vi "MonoSpec50 Goto.vi"(4 "PosDem":dbl caption="Position\nDemandée (nm)", 5 "Abort Ref":refnum<vi>, 6 "error in (no error)":errorcluster, 7 "PosAct":dbl caption="Position\nActuelle (nm)", 8 "Moving Ref":refnum<vi>, 9 "Ask Act Pos":bool=TRUE caption="Demander la \nposition actuelle (nm)") -> (0 "error out":errorcluster, 1 "PosAct Out":dbl caption="Position\nActuelle (nm)")   [LabVIEW 2012]
doc: "Ce Vi permet l'envoie de commande de déplacement au contrôlleur de moteur du monochromateur MonoSpec50."
uses:
  <userlib>/Monospec 50/MonoSpec50 Goto States.ctl
panel:
  out "large":bool
  out "NegPulse":bool
  out "Blocs":dbl
  in  "Abort":bool
  out "NbPas":dbl
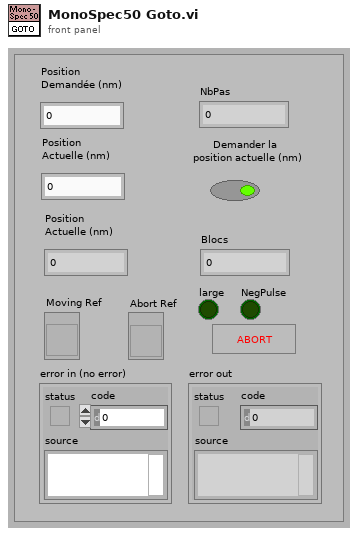
[diagram p1: front panel]
types:
  T1 = typedef "MonoSpec50 Goto States.ctl" = enum16{"PosLargeMov", "Back1Large", "largeMoveBloc", "Init Wavelenght", "Find Direction", "Send Pulses", "NegLargeMove", "End"}
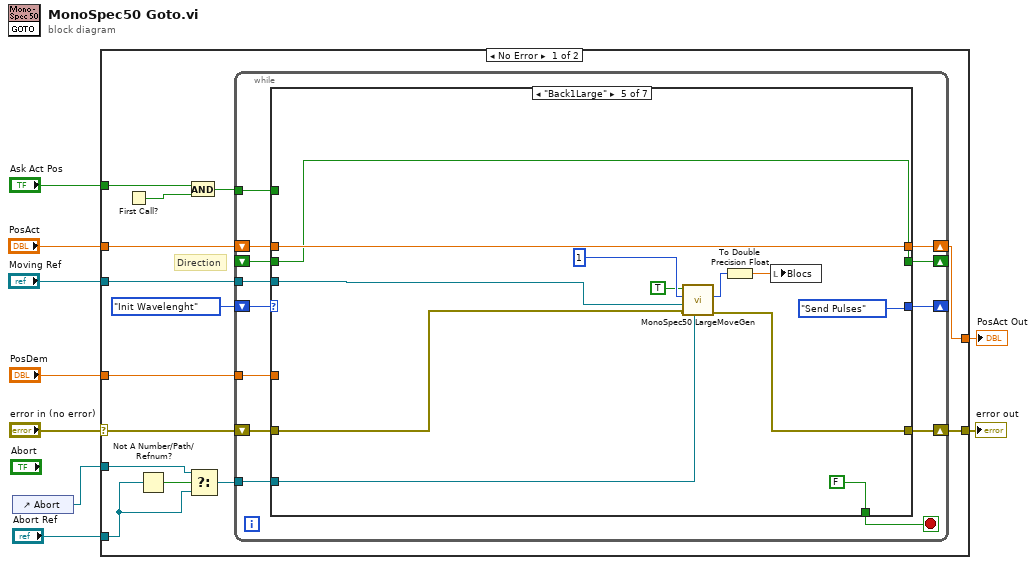
[diagram p0: block diagram]
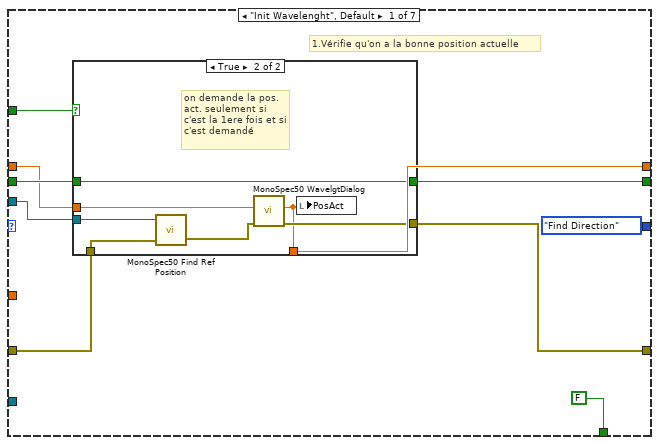
[diagram p2: hidden frame]
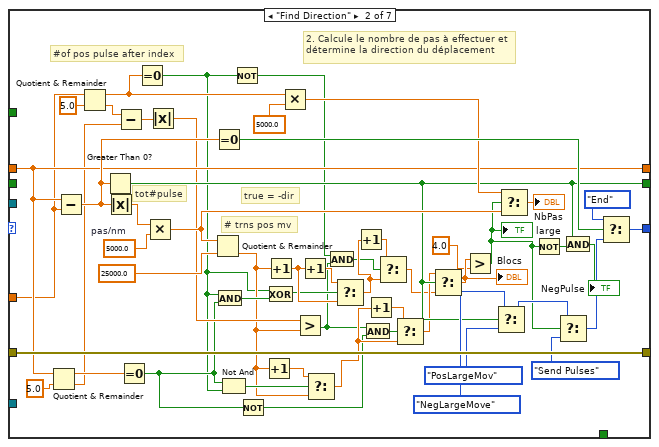
[diagram p4: hidden frame]
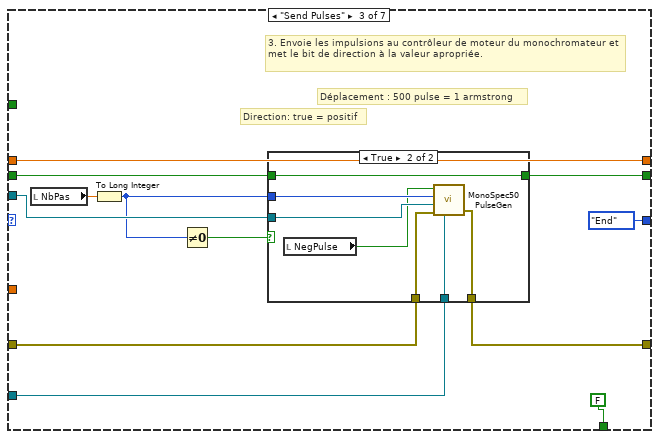
[diagram p5: hidden frame]
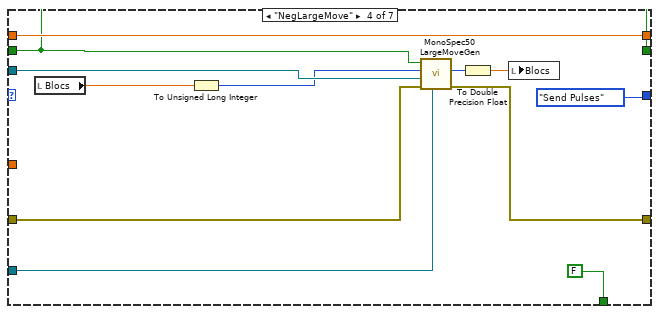
[diagram p7: hidden frame]
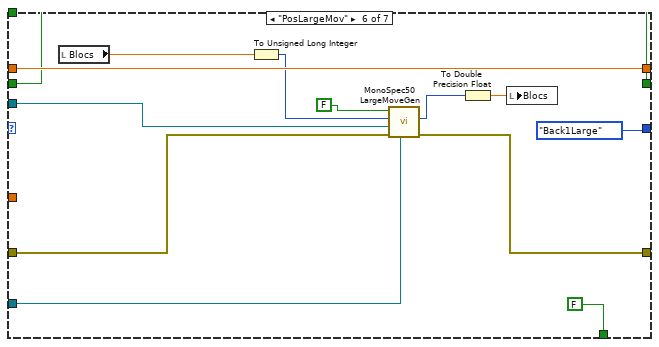
[diagram p8: hidden frame]
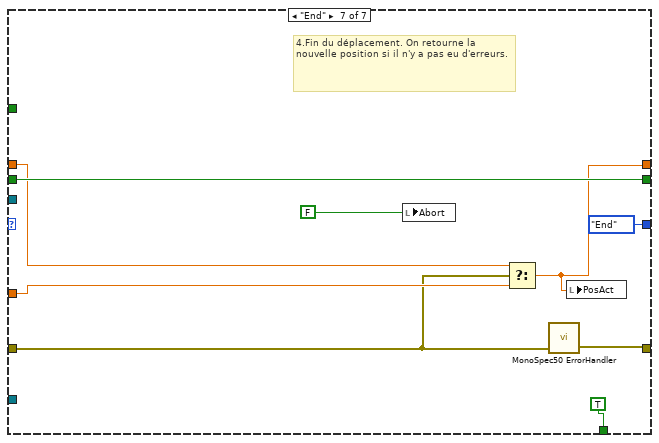
[diagram p9: hidden frame]
diagram:
  n1 = control-ref of="Abort"() -> (w1:refnum<vi>)
  n2 = case shown="No Error" "error in (no error)" {
    selector: "error in (no error)" -> [w17 w178]
    tunnel: [w16 w178] -> w8
    tunnel: "PosAct" -> [w22 w177]
    tunnel: "Ask Act Pos" -> [w19 _]
    tunnel: "PosDem" -> [w18 _]
    tunnel: [w15 w177] -> w4
    tunnel: "Moving Ref" -> [w14 _]
    tunnel: "Abort Ref" -> [w12 _]
    tunnel: w1 -> [w11 _]
    frame No Error {
      # "Direction"
      n3 = First Call?() -> (First Call?: T/F=w20:bool)
      n4 = Not A Number/Path/Refnum?(number/path/refnum=w12) -> (NaN/Path/Refnum?=w13:bool)
      n5 = And(x=w19, y=w20) -> (x .and. y?=w21:bool)
      n6 = Select(t=w11, s=w13, f=w12) -> (s? t:f=w10:refnum<vi>)
      n7 = while {
        shift-right: [w32] -> _
        shift-left: MonoSpec50_Goto_States."Init Wavelenght" -> [w36]
        tunnel: w18 -> [w31]
        shift-right: [w30] -> _
        shift-left: _ -> [w29]
        shift-right: [w27] -> w16
        shift-left: w17 -> [w28]
        tunnel: w21 -> [w33]
        tunnel: w14 -> [w25]
        shift-right: [w26] -> w15
        shift-left: w22 -> [w34]
        tunnel: w10 -> [w24]
        stop <- w35 stop-if-true
        n8 = case shown="\"Back1Large\"" w36 {
          tunnel: [FALSE _ FALSE FALSE FALSE FALSE TRUE] -> w35
          tunnel: w34 -> [w39 w85 w115 w139 w152 w164 w173]
          tunnel: w33 -> [w45 _ _ _ _ _ _]
          tunnel: [MonoSpec50_Goto_States."Find Direction" w107 MonoSpec50_Goto_States."End" MonoSpec50_Goto_States."Send Pulses" MonoSpec50_Goto_States."Send Pulses" MonoSpec50_Goto_States."Back1Large" MonoSpec50_Goto_States."End"] -> w32
          tunnel: w31 -> [_ w81 _ _ _ _ w172]
          tunnel: [w42 w88 w112 w135 w148 w160 w176] -> w30
          tunnel: w29 -> [w43 _ w118 w135 w148 w160 w176]
          tunnel: w28 -> [w41 w105 w120 w138 w151 w163 w171]
          tunnel: [w40 w105 w119 w137 w150 w162 w170] -> w27
          tunnel: [w37 w85 w115 w139 w152 w164 w168] -> w26
          tunnel: w25 -> [w38 _ w114 w136 w149 w161 _]
          tunnel: w24 -> [_ _ w113 w134 w147 w159 _]
          frame "Init Wavelenght", Default {
            # "1.Vérifie qu'on a la bonne position actuelle"
            n9 = case shown="True" w45 {
              tunnel: w39 -> [w47 w54]
              tunnel: w43 -> [w49 w56]
              tunnel: [w49 w56] -> w42
              tunnel: w41 -> [w48 w53]
              tunnel: [w48 w55] -> w40
              tunnel: w38 -> [_ w51]
              tunnel: [w47 w50] -> w37
              frame False {
              }
              frame True {
                # "on demande la pos. act. seulement si c'est la 1ere fois et si c'est demandé"
                n10 = call <userlib>:"MonoSpec50 Find Ref Position.vi"("error in"=w53, "Moving Ref"=w51) -> ("error out"=w52:errorcluster)  [unwired: 1 in, 1 out]
                n11 = call <userlib>:"MonoSpec50 WavelgtDialog.vi"("error in (no error)"=w52, "PosAct"=w54) -> ("error out"=w55:errorcluster, "PosAct Out"=w50:dbl)  [unwired: 4 in]
                n12 = local write "PosAct"(w50) -> ()
              }
            }
          }
          frame "Find Direction" {
            w103 = 5000.0  # pas/nm
            # "# trns pos mv"
            # "tot#pulse"
            # "#of pos pulse after index"
            # "2. Calcule le nombre de pas à effectuer et détermine la direction du déplacement"
            # "true = -dir"
            n13 = Quotient & Remainder(x=w85, y=5.0) -> (x-y*floor(x/y)=w93:dbl, floor(x/y)=w74:dbl)
            n14 = Subtract(x=w85, y=w81) -> (x-y=w106:dbl)
            n15 = Quotient & Remainder(x=w81, y=5.0) -> (x-y*floor(x/y)=w90:dbl, floor(x/y)=w75:dbl)
            n16 = Greater Than 0?(x=w106) -> (x > 0?=w88:bool)
            n17 = Absolute Value(x=w106) -> (abs(x)=w104:dbl)
            n18 = Subtract(x=w75, y=w74) -> (x-y=w73:dbl)
            n19 = Equal To 0?(x=w93) -> (x = 0?=w67:bool)
            n20 = Equal To 0?(x=w90) -> (x = 0?=w58:bool)
            n21 = Multiply(x=w104, y=w103) -> (x*y=w100:dbl)
            n22 = Absolute Value(x=w73) -> (abs(x)=w71:dbl)
            n23 = Quotient & Remainder(x=w100, y=25000.0) -> (floor(x/y)=w65:dbl)  [unwired: 1 out]
            n24 = Equal To 0?(x=w106) -> (x = 0?=w109:bool)
            n25 = And(x=w58, y=w67) -> (x .and. y?=w72:bool)
            n26 = Not And(1:w58, 2:w67) -> (0:w79:bool)
            n27 = Not(x=w58) -> (.not. x?=w57:bool)
            n28 = Not(x=w67) -> (.not. x?=w66:bool)
            n29 = Increment(x=w65) -> (x+1=w77:dbl)
            n30 = Increment(x=w65) -> (x+1=w84:dbl)
            n31 = Exclusive Or(1:w72, 2:w58) -> (0:w82:bool)
            n32 = Multiply(x=w90, y=5000.0) -> (x*y=w95:dbl)
            n33 = Greater?(x=w71, y=w65) -> (0:w60:bool)
            n34 = Increment(x=w84) -> (x+1=w83:dbl)
            n35 = Select(t=w77, s=w79, f=w65) -> (s? t:f=w70:dbl)
            n36 = And(x=w57, y=w60) -> (x .and. y?=w59:bool)
            n37 = Select(t=w83, s=w82, f=w84) -> (s? t:f=w61:dbl)
            n38 = Increment(x=w61) -> (x+1=w62:dbl)
            n39 = And(x=w60, y=w66) -> (x .and. y?=w69:bool)
            n40 = Increment(x=w70) -> (x+1=w64:dbl)
            n41 = Select(t=w62, s=w59, f=w61) -> (s? t:f=w63:dbl)
            n42 = Select(t=w64, s=w69, f=w70) -> (s? t:f=w68:dbl)
            n43 = Select(t=w68, s=w88, f=w63) -> (s? t:f=w78:dbl)
            "Blocs" <- w78
            n44 = Greater?(x=w78, y=4.0) -> (0:w80:bool)
            "large" <- w80
            n45 = Select(t=MonoSpec50_Goto_States."NegLargeMove", s=w88, f=MonoSpec50_Goto_States."PosLargeMov") -> (s? t:f=w97:T1)
            n46 = Select(t=w95, s=w80, f=w100) -> (s? t:f=→"NbPas":dbl)
            n47 = Not(x=w80) -> (.not. x?=w89:bool)
            n48 = Select(t=w97, s=w80, f=MonoSpec50_Goto_States."Send Pulses") -> (s? t:f=w101:T1)
            n49 = And(x=w88, y=w89) -> (x .and. y?=→"NegPulse":bool)
            n50 = Select(t=MonoSpec50_Goto_States."End", s=w109, f=w101) -> (s? t:f=w107:T1)
          }
          frame "Send Pulses" {
            # "Direction: true = positif"
            # "Déplacement : 500 pulse = 1 armstrong"
            # "3. Envoie les impulsions au contrôleur de moteur du monochromateur et met le bit de direction à la valeur apropriée."
            n51 = local read "NbPas"() -> (w121:dbl)
            n52 = To Long Integer(number=w121) -> (32bit integer=w111:i32)
            n53 = Not Equal To 0?(x=w111) -> (x != 0?=w110:bool)
            n54 = case shown="True" w110 {
              tunnel: w120 -> [w122 w130]
              tunnel: [w122 w129] -> w119
              tunnel: w118 -> [w123 w125]
              tunnel: w111 -> [_ w128]
              tunnel: w114 -> [_ w127]
              tunnel: w113 -> [_ w126]
              tunnel: [w123 w125] -> w112
              frame False {
              }
              frame True {
                n55 = local read "NegPulse"() -> (w124:bool)
                n56 = call <userlib>:"MonoSpec50 PulseGen.vi"("Abort Ref"=w126, "error in"=w130, "Moving Ref"=w127, "nb pulse"=w128, "Directions"=w124) -> ("error out"=w129:errorcluster)  [unwired: 4 in, 1 out]
              }
            }
          }
          frame "NegLargeMove" {
            n57 = local read "Blocs"() -> (w141:dbl)
            n58 = To Unsigned Long Integer(number=w141) -> (unsigned 32bit integer=w131:u32)
            n59 = call <userlib>:"MonoSpec50 LargeMoveGen.vi"("Abort Ref"=w134, "error in"=w138, "Moving Ref"=w136, "Turns"=w131, "Directions"=w135) -> ("error out"=w137:errorcluster, "Compte"=w133:u32)  [unwired: 1 in, 1 out]
            n60 = To Double Precision Float(number=w133) -> (double precision float=w132:dbl)
            n61 = local write "Blocs"(w132) -> ()
          }
          frame "Back1Large" {
            n62 = call <userlib>:"MonoSpec50 LargeMoveGen.vi"("Abort Ref"=w147, "error in"=w151, "Moving Ref"=w149, "Turns"=u32 1, "Directions"=TRUE) -> ("error out"=w150:errorcluster, "Compte"=w146:u32)  [unwired: 1 in, 1 out]
            n63 = To Double Precision Float(number=w146) -> (double precision float=w145:dbl)
            n64 = local write "Blocs"(w145) -> ()
          }
          frame "PosLargeMov" {
            n65 = local read "Blocs"() -> (w166:dbl)
            n66 = To Unsigned Long Integer(number=w166) -> (unsigned 32bit integer=w155:u32)
            n67 = call <userlib>:"MonoSpec50 LargeMoveGen.vi"("Abort Ref"=w159, "error in"=w163, "Moving Ref"=w161, "Turns"=w155, "Directions"=FALSE) -> ("error out"=w162:errorcluster, "Compte"=w158:u32)  [unwired: 1 in, 1 out]
            n68 = To Double Precision Float(number=w158) -> (double precision float=w157:dbl)
            n69 = local write "Blocs"(w157) -> ()
          }
          frame "End" {
            # "4.Fin du déplacement. On retourne la nouvelle position si il n'y a pas eu d'erreurs."
            n70 = local write "Abort"(FALSE ("Abort")) -> ()
            n71 = Select(t=w173, s=w171, f=w172) -> (s? t:f=w168:dbl)
            n72 = call <userlib>:"MonoSpec50 ErrorHandler.vi"("error in (no error)"=w171) -> ("error out"=w170:errorcluster)  [unwired: 1 in, 1 out]
            n73 = local write "PosAct"(w168) -> ()
          }
        }
      }
    }
    frame Error {
    }
  }
  "error out" <- w8
  "PosAct Out" <- w4
